vi "data_to_parser.vi"(6 "port":u16, 7 "connection ID out":refnum<k16>, 8 "error in (no error)":errorcluster, 9 "address":u32, 10 "udp message":string, 11 "UDP_receiver in":refnum<class "UDP_receiver.lvclass">) -> (0 "error out":errorcluster, 3 "UDP_receiver out":refnum<class "UDP_receiver.lvclass">)   [LabVIEW 2025, in "UDP_receiver.lvlib" / "UDP_receiver.lvclass"]
uses:
  UDP_receiver.lvclass
  UDP_receiver.lvclass/UDP_receiver.ctl
  Send Notification Messages/send response Msg/send response Msg.lvclass/send response Msg.ctl
  <vilib>/ActorFramework/Message Enqueuer/Message Enqueuer.lvclass/Message Enqueuer.ctl
  <vilib>/ActorFramework/Message Enqueuer/Enqueue.vi
  Send Notification Messages/send response Msg/send response Msg.lvclass
  Applications/National Instruments/LabVIEW 2025 64-bit/vi.lib/ActorFramework/Message/Message.lvclass
  <vilib>/ActorFramework/Message Priority Queue/Priority Enqueue.vi
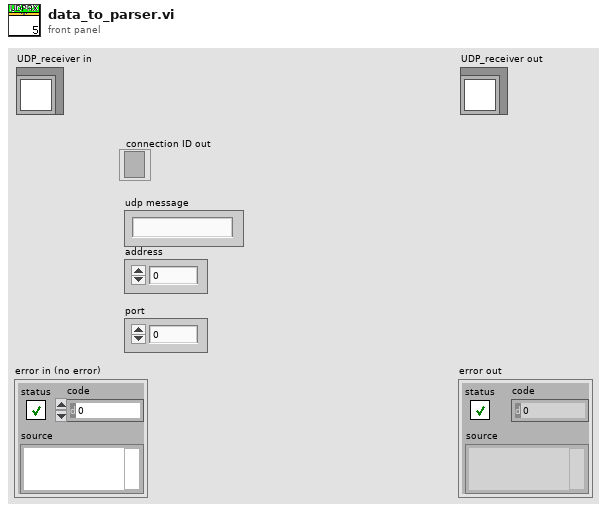
[diagram p1: front panel]
types:
  T1 = map{string, refnum<class "Message Enqueuer.lvclass">}
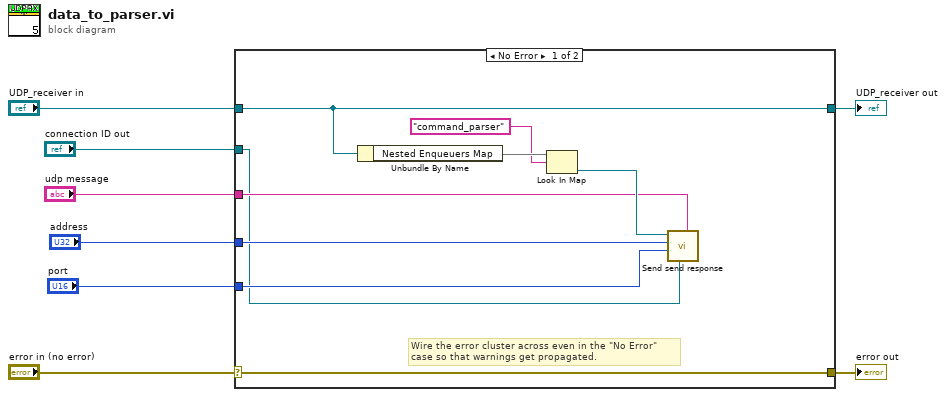
[diagram p0: block diagram]
diagram:
  n1 = case shown="No Error" "error in (no error)" {
    selector: "error in (no error)" -> [w17 w19]
    tunnel: [w17 w19] -> w7
    tunnel: [w16 w18] -> w5
    tunnel: "UDP_receiver in" -> [w16 w18]
    tunnel: "connection ID out" -> [w9 _]
    tunnel: "udp message" -> [w12 _]
    tunnel: "address" -> [w11 _]
    tunnel: "port" -> [w10 _]
    frame No Error {
      # "Wire the error cluster across even in the \"No Error\"\ncase so that warnings get propagated."
      n2 = Unbundle By Name(w16) -> ("Nested Enqueuers Map"=w15:T1)
      n3 = Look In Map(map=w15, key="command_parser") -> (value=w13:refnum<class "Message Enqueuer.lvclass">)  [unwired: 1 in, 1 out]
      n4 = call "Send send response.vi"("udp message"=w12, "connection ID out"=w9, "port"=w10, "address"=w11, "Message Enqueuer"=w13) -> ()  [unwired: 5 in, 2 out]
    }
    frame Error {
    }
  }
  "error out" <- w7
  "UDP_receiver out" <- w5
